vi "Read Configuration Parameters.vi"(8 "error in (no error)":errorcluster, 10 "refnum":T1, 11 "Example Configuration Dialog in":refnum<class "Slave Config.lvclass">) -> (0 "error out":errorcluster, 2 "refnum out":T1, 3 "Example Configuration Dialog out":refnum<class "Slave Config.lvclass">)   [LabVIEW 2016, in "Slave Config.lvclass"]
uses:
  <userlib>/Common Components/Slave Configuration/Slave Config.lvclass
  <vilib>/Utility/config.llb/Config Data RefNum.ctl
  <userlib>/Common Components/Slave Configuration/Slave Config.lvclass/Slave Config.ctl
  <userlib>/Configuration Dialog Actor/Configuration.lvclass
  <vilib>/Utility/config.llb/NI_LVConfig.lvlib
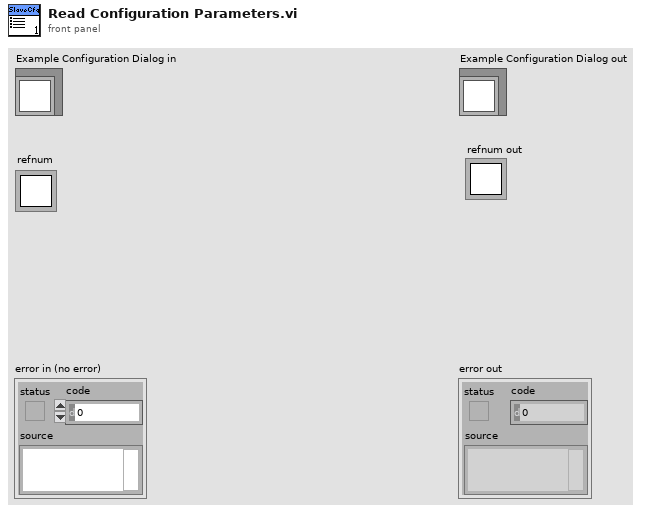
[diagram p1: front panel]
types:
  T1 = typedef "NI_LVConfig.lvlib/Config Data RefNum.ctl" = refnum<k1>
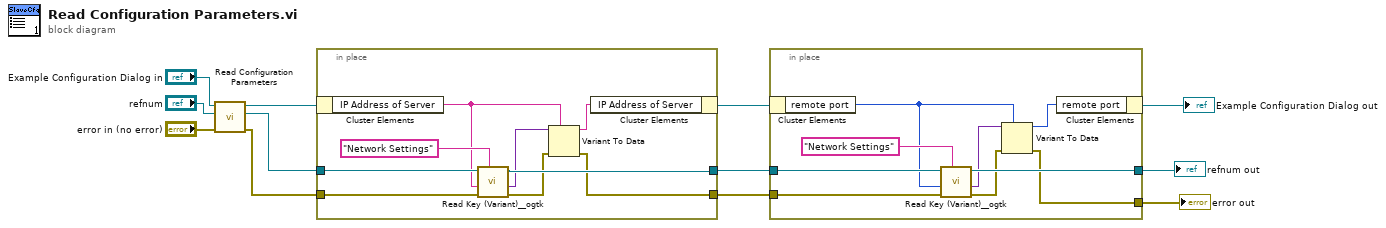
[diagram p0: block diagram]
diagram:
  n1 = call-parent "Read Configuration Parameters.vi"("error in (no error)"="error in (no error)", "refnum"="refnum", "Configuration in"="Example Configuration Dialog in") -> ("error out"=w3:errorcluster, "refnum out"=w6:T1, "Configuration out"=w8:refnum<class "Slave Config.lvclass">)  [unwired: 6 in]
  n2 = in-place "In Place Element Structure" {
    in-place-border: w6 -> [w21]
    in-place-border: [w20] -> w5
    in-place-border: [w15] -> w4
    in-place-border: w3 -> [w14]
    n3 = in-place-cluster #1(w8) -> ("IP Address of Server"=w13:string)
    n4 = call <userlib>:"Read Key (Variant)__ogtk.vi"("section"="Network Settings", "error in (no error)"=w14, "type"=w13, "refnum"=w21) -> ("error out"=w16:errorcluster, "key-value"=w17:variant, "refnum out"=w20:T1)  [unwired: 4 in, 1 out]
    n5 = Variant To Data(error in=w16, type=w13, Variant=w17) -> (data=w18:string, error out=w15:errorcluster)
    n6 = in-place-cluster #1("IP Address of Server"=w18) -> (w9:refnum<class "Slave Config.lvclass">)
  }
  n7 = in-place "In Place Element Structure" {
    in-place-border: [w29] -> w2
    in-place-border: w5 -> [w30]
    in-place-border: w4 -> [w24]
    in-place-border: [w22] -> w1
    n8 = in-place-cluster #2(w9) -> ("remote port"=w25:u16)
    n9 = call <userlib>:"Read Key (Variant)__ogtk.vi"("section"="Network Settings", "error in (no error)"=w24, "type"=w25, "refnum"=w30) -> ("error out"=w23:errorcluster, "key-value"=w27:variant, "refnum out"=w29:T1)  [unwired: 4 in, 1 out]
    n10 = Variant To Data(error in=w23, type=w25, Variant=w27) -> (data=w26:u16, error out=w22:errorcluster)
    n11 = in-place-cluster #2("remote port"=w26) -> (→"Example Configuration Dialog out":refnum<class "Slave Config.lvclass">)
  }
  "error out" <- w1
  "refnum out" <- w2
